vi "GenerateFullPressureSequence.vi"(9 "Mix Cluster":T1={"Ratio"=[0.6, 0.5], "Mix 2"=[12, 12], "Mix 1"=[0, 1]} {"Mix 1" items=["A1"=0, "A2"=1, "A3"=2, "A4"=3, "A5"=12]; "Mix 2" items=["B5"=8, "B6"=9, "B7"=10, "B8"=11, "A5"=12]}, 10 "Pressure For Mix 2":dbl[](array[numeric]), 11 "Pressure For Mix 1":dbl[](array[numeric])) -> (3 "Pressure Sequence (Ch 2-4)":dbl[][](array[numeric]))   [LabVIEW 2016]
panel:
  out "Array 2":i32[](array[numeric])
  out "Array":i32[](array[numeric])
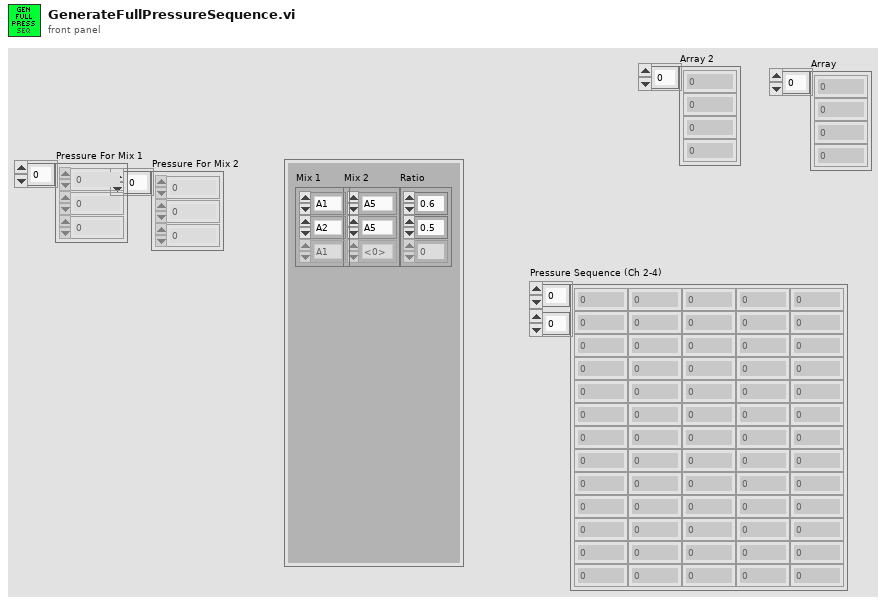
[diagram p1: front panel]
types:
  T1 = cluster{"Ratio":dbl[], "Mix 2":u16[], "Mix 1":u16[]}
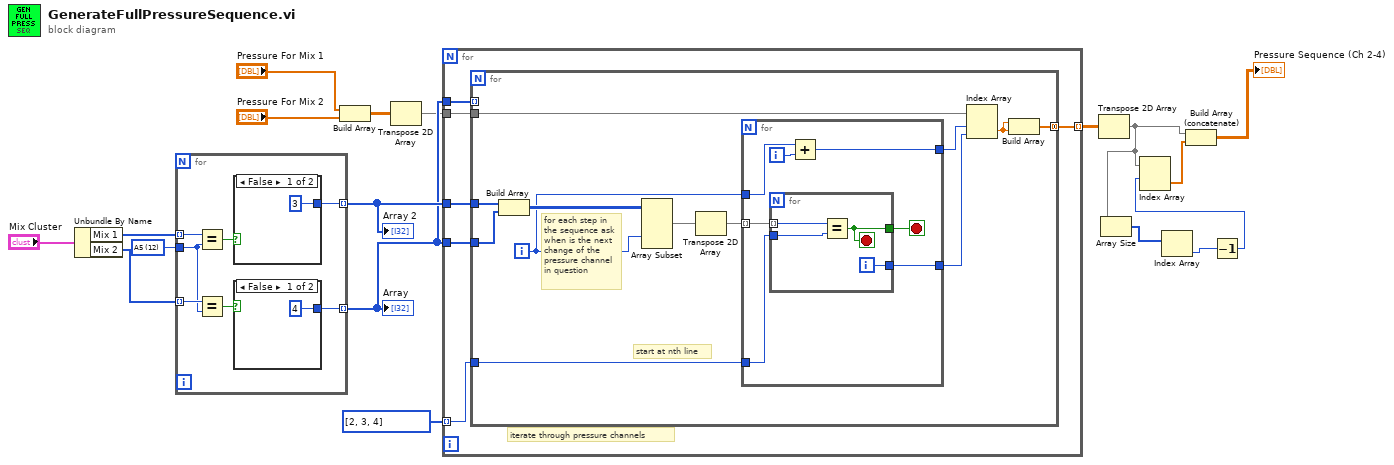
[diagram p0: block diagram]
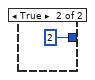
[diagram p2: hidden frame]
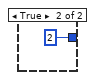
[diagram p3: hidden frame]
diagram:
  w15 = u16 12 items=["A1", "A2", "A3", "A4", "B1", "B2", "B3", "B4", "B5", "B6", "B7", "B8", "A5", "A6", "A7", "A8"] ("Mix Water Valve")
  n1 = Unbundle By Name("Mix Cluster") -> ("Mix 1"=w17:u16[], "Mix 2"=w16:u16[])
  n2 = for {
    tunnel: w17 -> [w23] mode=indexing
    tunnel: w16 -> [w25] mode=indexing
    tunnel: w15 -> [w24]
    tunnel: [w21] -> w14 mode=indexing
    tunnel: [w19] -> w9 mode=indexing
    n3 = Equal?(x=w23, y=w24) -> (x = y?=w22:bool)
    n4 = Equal?(x=w25, y=w24) -> (x = y?=w20:bool)
    n5 = case shown="False" w22 {
      tunnel: [3 2] -> w21
      frame False {
      }
      frame True {
      }
    }
    n6 = case shown="False" w20 {
      tunnel: [4 2] -> w19
      frame False {
      }
      frame True {
      }
    }
  }
  "Array" <- w9
  "Array 2" <- w14
  n7 = Build Array("Pressure For Mix 1", "Pressure For Mix 2") -> (w11:dbl[][])
  n8 = Transpose 2D Array(2D array=w11) -> (transposed array=w7:dbl[][])
  n9 = for {
    tunnel: w9 -> [w30]
    tunnel: w14 -> [w35]
    tunnel: w7 -> [w34]
    tunnel: [w33] -> w8 mode=indexing
    tunnel: i32[] [2, 3, 4] -> [w32] mode=indexing
    tunnel: w9 -> [w31]
    # "iterate through pressure channels"
    n10 = for {
      tunnel: w31 -> [w47]
      tunnel: w35 -> [w46]
      tunnel: w32 -> [w45]
      tunnel: w34 -> [w42]
      tunnel: [w36] -> w33 mode=concatenating
      tunnel: w30 -> [_] mode=indexing
      i -> [w38]
      # "for each step in the sequence ask when is the next change of the pressure channel in question"
      # "start at nth line"
      n11 = Build Array(w46, w47) -> (w44:i32[][])
      n12 = Array Subset(array=w44, index (col)=w38) -> (w43:i32[][])  [unwired: 3 in]
      n13 = Transpose 2D Array(2D array=w43) -> (transposed array=w39:i32[][])
      n14 = for {
        tunnel: w39 -> [w54] mode=indexing
        tunnel: w45 -> [w53]
        tunnel: [w51] -> w40
        tunnel: [w49] -> w41
        tunnel: w38 -> [w48]
        i -> [w50]
        stop <- w52 stop-if-true
        n15 = for {
          tunnel: w54 -> [w57] mode=indexing
          tunnel: w53 -> [w58]
          tunnel: [w56] -> w52
          tunnel: [w55] -> w51
          i -> [w55]
          stop <- w56 stop-if-true
          n16 = Equal?(x=w57, y=w58) -> (x = y?=w56:bool)
        }
        n17 = Add(x=w48, y=w50) -> (x+y=w49:i32)
      }
      n18 = Index Array(array=w42, index (row)=w41, index (col)=w40) -> (element=w37:dbl)
      n19 = Build Array(w37, w37) -> (w36:dbl[])
    }
  }
  n20 = Transpose 2D Array(2D array=w8) -> (transposed array=w2:dbl[][])
  n21 = Array Size(array=w2) -> (size(s)=w6:i32[])
  n22 = Index Array(array=w6) -> (element=w5:i32)  [unwired: 1 in]
  n23 = Decrement(x=w5) -> (x-1=w4:i32)
  n24 = Index Array(array=w2, index (row)=w4) -> (element=w3:dbl[])  [unwired: 1 in]
  n25 = Build Array (concatenate)(w2, w3) -> (→"Pressure Sequence (Ch 2-4)":dbl[][])
